vi "Ball Shooter Controller.vi"(8 "error in":errorcluster) -> ()   [LabVIEW 2016]
doc: "This VI executes continuously carrying out the current operation and responding to updates or new operations. It will often contain the timing or control code that is difficult to place directly in TeleOp. This VI generally opens all sensors and motors and isolates the rest of the robot code from knowing how the operations are carried out."
uses:
  Ball Shooter Setpoints.ctl
  Ball Shooter Operations.ctl
  <vilib>/Rock Robotics/WPI/ThirdParty/CanMotor/TalonSRX/WPI_CANTalonSRX_APIFeedbackSelect.ctl
  <vilib>/Rock Robotics/WPI/ThirdParty/CanMotor/TalonSRX/WPI_CANTalonSRX_APIControlMode.ctl
  <vilib>/Rock Robotics/WPI/SerialPort/WPI_SerialPort.ctl
  Ball Shooter Global.vi
panel:
  in  "Act":dbl
  out "Waveform Chart":cluster{"Act":dbl, "Encoder Velocity":dbl}(graph)
  in  "Cycle Period":dbl=1000.0
  in  "Cycle":bool
  out "Current\nCmd":string
  # "Tip: It may be helpful to observe inputs and sensor values.\nYou may also want to display tuning or debugging controls."
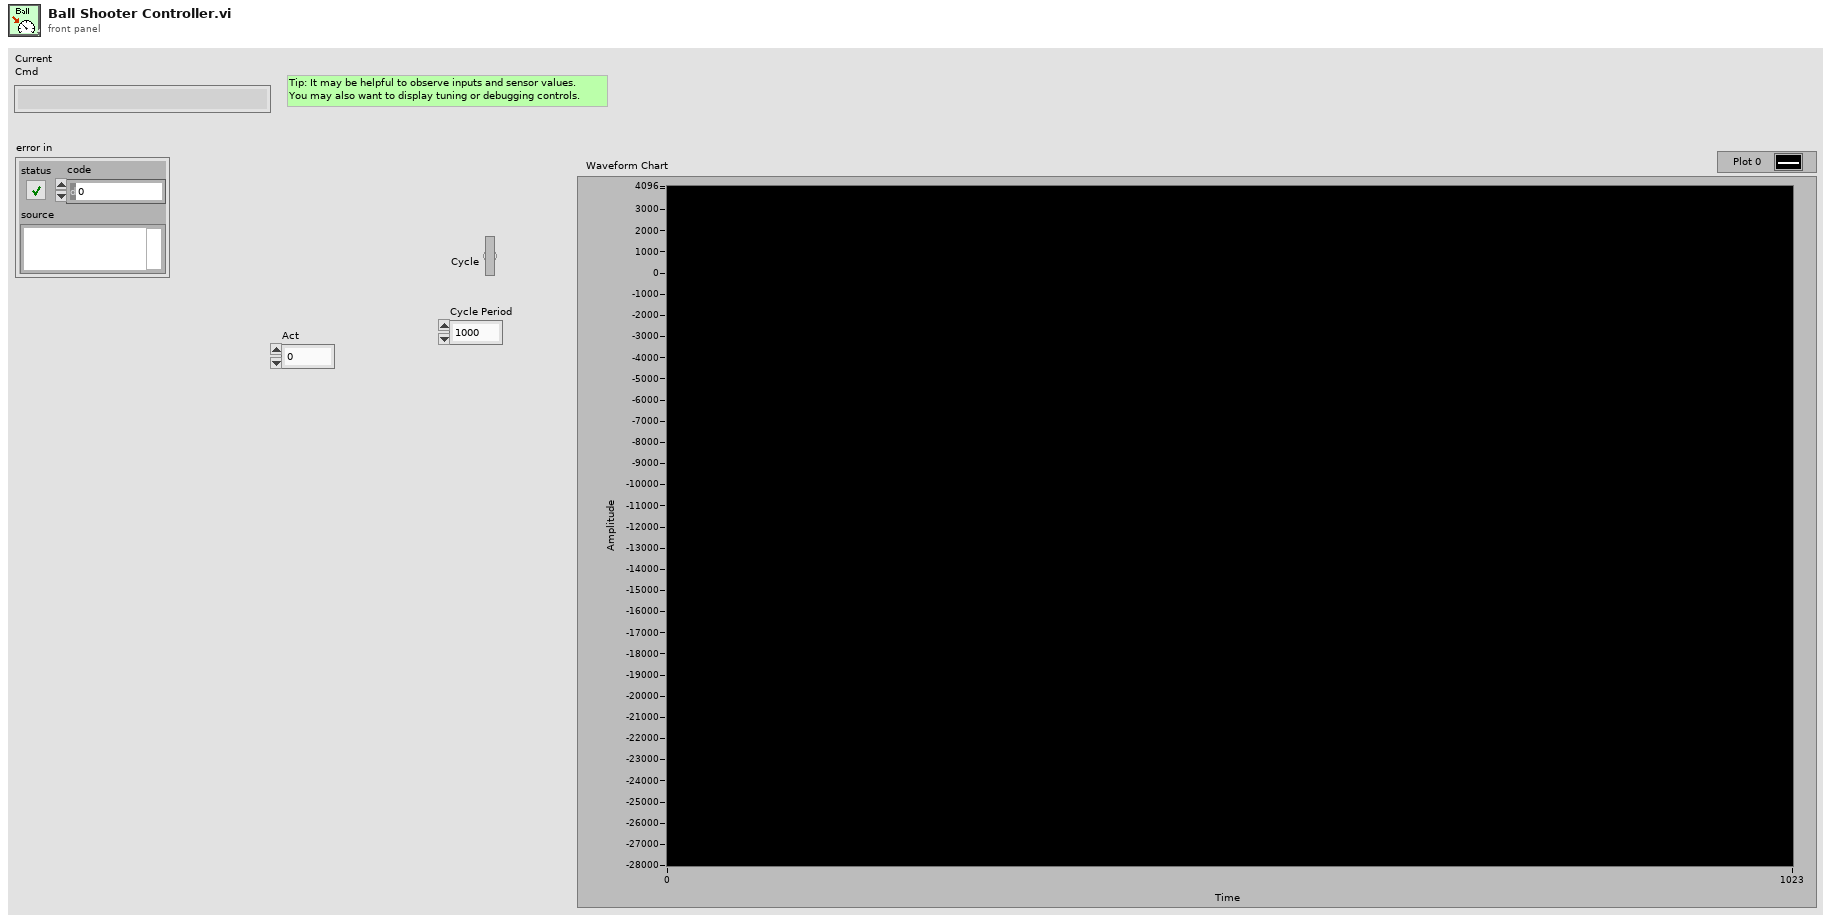
[diagram p1: front panel]
types:
  T1 = typedef "WPI_SerialPort.ctl" = enum16{"Onboard RS-232", "MXP TTL", "USB 1", "USB 2"}
  T2 = typedef "WPI_CANTalonSRX_APIControlMode.ctl" = enum8{"Percent VBus", "Speed", "Position", "Slave", "Unchanged / Invalid", "Voltage Compensation", "Current", "Motion Profile", "Motion Magic"}
  T3 = typedef "WPI_CANTalonSRX_APIFeedbackSelect.ctl" = enum16{"Digital Quadrature Encoder", "Analog Potentiometer", "Analog Encoder", "Count on Quad-A (Rising-Edge)", "Count on Quad-A (Falling-Edge)", "CTR Magnetic Enc (Absolute)", "CTR Magnetic Enc (Relative)", "Pulse Width"}
  T4 = typedef "Ball Shooter Setpoints.ctl" = cluster{"Operation":T5, "Setpoint":dbl, "Duration":dbl}
  T5 = typedef "Ball Shooter Operations.ctl" = enum16{"Reserve", "Read Current", "Immediate"}
  T6 = typedef "WPI_MotorControlDeviceRef.ctl" = cluster{"DeviceStatus":errorcluster, "Type":T7, "PWM":cluster{"PWM Channel":T8, "DeadBand":T9}, "CAN":cluster{"Device Number":u8, "SetOutput VI Ref":variant, "GetOutput VI Ref":variant, "Enable VI Ref":variant, "Disable VI Ref":variant, "Data":variant}, "Invert":bool}
  T7 = typedef "WPI_MotorControlType.ctl" = enum16{"PWM", "CAN"}
  T8 = typedef "FPGA_DIOPWMChannel.ctl" = enum8{"PWM 0", "PWM 1", "PWM 2", "PWM 3", "PWM 4", "PWM 5", "PWM 6", "PWM 7", "PWM 8", "PWM 9", "PWM MXP 0", "PWM MXP 1", "PWM MXP 2", "PWM MXP 3", "PWM MXP 4", "PWM MXP 5", "PWM MXP 6", "PWM MXP 7", "PWM MXP 8", "PWM MXP 9", "Invalid"}
  T9 = typedef "WPI_PWMDeadband.ctl" = cluster{"Name":string, "maxPositivePwm":i32, "minPositivePwm":i32, "centerPwm":i32, "maxNegativePwm":i32, "minNegativePwm":i32, "angularRange":u16}
  T10 = typedef "Command Status Info.ctl" = cluster{"Name":string, "Status":T11, "notifier out":T12}
  T11 = typedef "Completion Status.ctl" = enum16{"Successful", "Aborted", "Incomplete"}
  T12 = typedef "Completion Notifier.ctl" = refnum<notifier>
  T13 = cluster{"Default Command":T4, "Command Timing":cluster{"Start Time (ms)":u32, "Iterations":i32}, "Command Arguments":cluster{"Command Info":T10, "Description":string, "Default Command":T4, "notifier out":refnum<notifier>, "Subsystem Name":string}}
  T14 = typedef "WPI_SerialPortRef.ctl" = cluster{"DevStatus":errorcluster, "Serial Port Name":refnum<visa-resource-name>}
  T15 = typedef "WPI_CANTalonSRX_GlobalStatus.ctl" = cluster{"Applied Throttle":dbl, "Module Enabled":bool, "CAN Error":errorcluster, "Closed Loop Error":dbl, "Forward Limit Switch Closed":bool, "Reverse Limit Switch Closed":bool, "Sensor Position":dbl, "Sensor Velocity":dbl, "Current":dbl, "Sticky Fault - Over Temp":bool, "Sticky Fault - Under Voltage":bool, "Sticky Fault - Forward Limit":bool, "Sticky Fault - Reverse Limit":bool, "Sticky Fault - Forward Soft Limit":bool, "Sticky Fault - Reverse Soft Limit":bool, "Brake is Enabled":bool, "Encoder Position":dbl, "Encoder Velocity":dbl, "Encoder Index Count":dbl, "Encoder A Pin State":bool, "Encoder B Pin State":bool, "Encoder Index Pin State":bool, "Analog In":dbl, "Analog In Velocity":dbl, "Temperature (C)":dbl, "Battery Voltage":dbl, "Control 5 Is Supported":bool, "Current Profile Slot Select":dbl, "Pos Div 8":bool, "Vel Div 4":bool, "Pulse Width Position":i32, "Pulse Width Velocity":i32, "Pulse Width Rise To Rise (us)":i32, "Pulse Width Rise To Fall (us)":i32, "Mot Prof Active Is Under Run":bool, "Mot Prof Active Has Under Run":bool, "Mot Prof Active Is Last":bool, "Mot Prof Active Velocity Only":bool, "Mot Prof Active Is Valid":bool, "Mot Prof Buffer Is Full":bool, "Mot Prof Active Profile Slot Select":i32, "Mot Prof NextID":i32, "Mot Prof Count":i32, "Mot Prof Active Velocity":dbl, "Mot Prof Active Position":dbl, "Mot Prof Output Enable":i32}
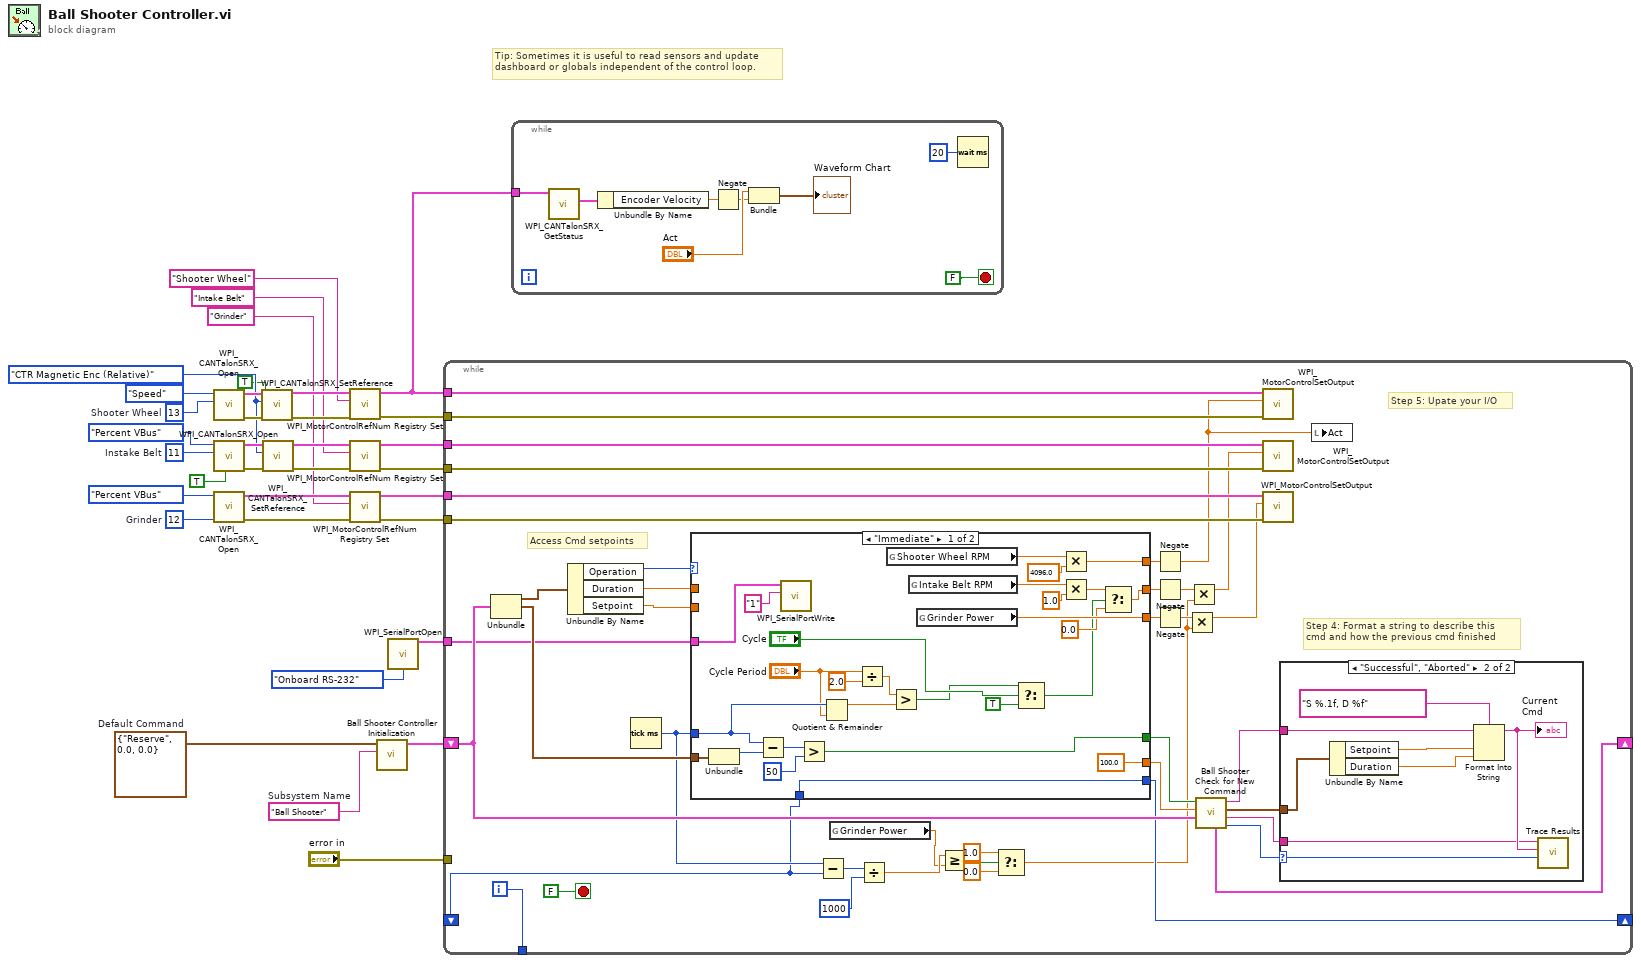
[diagram p0: block diagram]
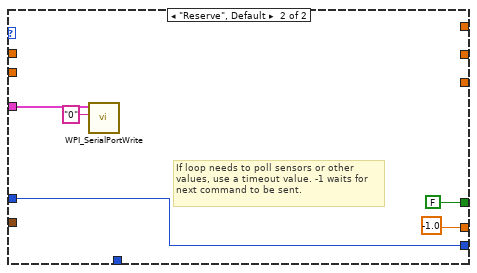
[diagram p3: hidden frame]
diagram:
  w21 = u8 12  # Grinder
  w23 = u8 11  # Instake Belt
  w24 = u8 13  # Shooter Wheel
  w26 = WPI_CANTalonSRX_APIFeedbackSelect."CTR Magnetic Enc (Relative)" ("Feedback Reference")
  w31 = T4 {"Operation"=enum."Reserve", "Setpoint"=0.0, "Duration"=0.0}  # Default Command
  w32 = "Ball Shooter"  # Subsystem Name
  # "Tip: Sometimes it is useful to read sensors and update\ndashboard or globals independent of the control loop."
  n1 = call <vilib>:"WPI_CANTalonSRX_Open.vi"("Device Number"=w24, "Control Mode"=WPI_CANTalonSRX_APIControlMode."Speed") -> ("error out"=w30:errorcluster, "CAN Talon SRX Ref"=w29:T6)  [unwired: 8 in]
  n2 = call <vilib>:"WPI_CANTalonSRX_Open.vi"("Invert"=TRUE, "Device Number"=w23, "Control Mode"=WPI_CANTalonSRX_APIControlMode."Percent VBus") -> ("error out"=w27:errorcluster, "CAN Talon SRX Ref"=w28:T6)  [unwired: 7 in]
  n3 = call <vilib>:"WPI_CANTalonSRX_Open.vi"("Device Number"=w21, "Control Mode"=WPI_CANTalonSRX_APIControlMode."Percent VBus") -> ("error out"=w12:errorcluster, "CAN Talon SRX Ref"=w14:T6)  [unwired: 8 in]
  n4 = call <vilib>:"WPI_CANTalonSRX_SetReference.vi"("error in (no error)"=w30, "Reverse Feedback Sensor"=TRUE, "Feedback Reference"=w26, "CAN Talon SRX Ref"=w29) -> ("error out"=w19:errorcluster, "CAN Talon SRX Ref"=w20:T6)  [unwired: 6 in]
  n5 = call <vilib>:"WPI_CANTalonSRX_SetReference.vi"("error in (no error)"=w27, "Feedback Reference"=w26, "CAN Talon SRX Ref"=w28) -> ("error out"=w11:errorcluster, "CAN Talon SRX Ref"=w16:T6)  [unwired: 7 in]
  n6 = call <vilib>:"WPI_MotorControlRefNum Registry Set.vi"("error in (no error)"=w19, "refnum name"="Shooter Wheel", "MotorControlDevRef"=w20) -> ("error out"=w17:errorcluster, "MotorControlDevRef"=w5:T6)  [unwired: 7 in]
  n7 = call <vilib>:"WPI_MotorControlRefNum Registry Set.vi"("error in (no error)"=w11, "refnum name"="Intake Belt", "MotorControlDevRef"=w16) -> ("error out"=w10:errorcluster, "MotorControlDevRef"=w15:T6)  [unwired: 7 in]
  n8 = call <vilib>:"WPI_MotorControlRefNum Registry Set.vi"("error in (no error)"=w12, "refnum name"="Grinder", "MotorControlDevRef"=w14) -> ("error out"=w9:errorcluster, "MotorControlDevRef"=w13:T6)  [unwired: 7 in]
  n9 = call "Ball Shooter Controller Initialization.vi"("Subsystem Name"=w32, "Default Command"=w31) -> ("Command Info"=w33:T13)  [unwired: 9 in]
  n10 = call <vilib>:"WPI_SerialPortOpen.vi"("Serial Port"=WPI_SerialPort."Onboard RS-232") -> ("SerialPortRef"=w2:T14)  [unwired: 13 in, 1 out]
  n11 = while {
    shift-right: [w67] -> _
    shift-left: w33 -> [w68]
    tunnel: [w74] -> _
    tunnel: "error in" -> [_]
    tunnel: w5 -> [w60]
    tunnel: w17 -> [w59]
    tunnel: w15 -> [w58]
    tunnel: w13 -> [w56]
    tunnel: w10 -> [w57]
    tunnel: w9 -> [w55]
    shift-right: [w47] -> _
    shift-left: _ -> [w48]
    tunnel: w2 -> [w35]
    i -> [w74]
    stop <- FALSE stop-if-true
    # "Step 5: Upate your I/O"
    # "Step 4: Format a string to describe this\ncmd and how the previous cmd finished"
    # "Access Cmd setpoints"
    n12 = Unbundle(w68) -> ("Default Command"=w73:T4, "Command Timing"=w70:cluster{"Start Time (ms)":u32, "Iterations":i32})  [unwired: 1 out]
    n13 = Unbundle By Name(w73) -> ("Operation"=w72:T5, "Duration"=w71:dbl, "Setpoint"=w69:dbl)
    n14 = Tick Count (ms)() -> (millisecond timer value=w49:u32)
    n15 = case shown="\"Immediate\"" w72 {
      tunnel: [100.0 -1.0] -> w65
      tunnel: [w105 FALSE ("ignore previous (F)")] -> w66
      tunnel: w70 -> [w106 _]
      tunnel: w71 -> [_ _]
      tunnel: w49 -> [w98 w113]
      tunnel: w69 -> [_ _]
      tunnel: [w99 _] -> w54
      tunnel: [w92 _] -> w53
      tunnel: [w104 _] -> w52
      tunnel: w48 -> [w86 _]
      tunnel: [w86 w113] -> w47
      tunnel: w35 -> [w85 w112]
      frame "Immediate" {
        n16 = Unbundle(w106) -> ("Start Time (ms)"=w109:u32)  [unwired: 1 out]
        n17 = Subtract(x=w98, y=w109) -> (x-y=w108:u32)
        n18 = call <vilib>:"WPI_SerialPortWrite.vi"("Buffer"="1", "SerialPortRef"=w85) -> ()  [unwired: 7 in, 3 out]
        n19 = Greater?(x=w108, y=u8 50 ("Left Motor")) -> (0:w105:bool)
        n20 = Quotient & Remainder(x=w98, y="Cycle Period") -> (x-y*floor(x/y)=w94:dbl)  [unwired: 1 out]
        n21 = Divide(x="Cycle Period", y=2.0) -> (x/y=w95:dbl)
        n22 = global read "Ball Shooter Global.vi" "Shooter Wheel RPM"() -> (w100:dbl)
        n23 = Greater?(x=w95, y=w94) -> (0:w88:bool)
        n24 = global read "Ball Shooter Global.vi" "Intake Belt RPM"() -> (w103:dbl)
        n25 = global read "Ball Shooter Global.vi" "Grinder Power"() -> (w104:dbl)
        n26 = Select(t=w88, s="Cycle", f=TRUE) -> (s? t:f=w90:bool)
        n27 = Multiply(x=w100, y=4096.0) -> (x*y=w99:dbl)
        n28 = Multiply(x=w103, y=1.0) -> (x*y=w93:dbl)
        n29 = Select(t=w93, s=w90, f=0.0) -> (s? t:f=w92:dbl)
      }
      frame "Reserve", Default {
        # "If loop needs to poll sensors or other\nvalues, use a timeout value. -1 waits for\nnext command to be sent."
        n30 = call <vilib>:"WPI_SerialPortWrite.vi"("Buffer"="0", "SerialPortRef"=w112) -> ()  [unwired: 7 in, 3 out]
      }
    }
    n31 = Subtract(x=w49, y=w48) -> (x-y=w46:u32)
    n32 = global read "Ball Shooter Global.vi" "Grinder Power"() -> (w43:dbl)
    n33 = Divide(x=w46, y=u32 1000) -> (x/y=w44:dbl)
    n34 = Greater Or Equal?(x=w44, y=w43) -> (x >= y?=w42:bool)
    n35 = Select(t=1.0, s=w42, f=0.0) -> (s? t:f=w36:dbl)
    n36 = Negate(x=w54) -> (-x=w50:dbl)
    n37 = Negate(x=w53) -> (-x=w51:dbl)
    n38 = Negate(x=w52) -> (-x=w38:dbl)
    n39 = Multiply(x=w38, y=w36) -> (x*y=w37:dbl)
    n40 = Multiply(x=w51, y=w36) -> (x*y=w39:dbl)
    n41 = call "Ball Shooter Check for New Command.vi"("Current Command"=w68, "Wait time (ms)"=w65, "Finished?"=w66) -> ("Completion"=w61:T11, "Subsystem Name"=w62:string, "Current Command"=w63:T4, "Initial Trace String"=w64:string, "NextCommand"=w67:T13)  [unwired: 4 in]
    n42 = call <vilib>:"WPI_MotorControlSetOutput.vi"("error in (no error)"=w59, "Output"=w50, "MotorControlDevRef"=w60) -> ()  [unwired: 6 in, 3 out]
    n43 = call <vilib>:"WPI_MotorControlSetOutput.vi"("error in (no error)"=w57, "Output"=w39, "MotorControlDevRef"=w58) -> ()  [unwired: 6 in, 3 out]
    n44 = call <vilib>:"WPI_MotorControlSetOutput.vi"("error in (no error)"=w55, "Output"=w37, "MotorControlDevRef"=w56) -> ()  [unwired: 6 in, 3 out]
    n45 = case shown="\"Successful\", \"Aborted\"" w61 {
      selector: w61 -> [_ w83]
      tunnel: w64 -> [_ w79]
      tunnel: w63 -> [_ w80]
      tunnel: w62 -> [_ w76]
      frame "Incomplete", Default {
        # "Continuing current command"
      }
      frame "Successful", "Aborted" {
        # "Report and setup for next command"
        n46 = Unbundle By Name(w80) -> ("Setpoint"=w82:dbl, "Duration"=w77:dbl)
        n47 = Format Into String(format string="S %.1f, D %f", initial string=w79, w82, w77) -> (resulting string=w78:string)  [unwired: 1 in, 1 out]
        "Current\nCmd" <- w78
        n48 = call <vilib>:"Trace Results.vi"("Status of previous command"=w83, "Description"=w78, "Subsystem"=w76) -> ()  [unwired: 9 in]
      }
    }
    n49 = local write "Act"(w50) -> ()
  }
  n50 = while {
    tunnel: w5 -> [w121]
    stop <- FALSE stop-if-true
    n51 = call <vilib>:"WPI_CANTalonSRX_GetStatus.vi"("CAN Talon SRX Ref"=w121) -> ("Talon SRX Status"=w120:T15)  [unwired: 8 in, 2 out]
    n52 = Unbundle By Name(w120) -> ("Encoder Velocity"=w119:dbl)
    n53 = Negate(x=w119) -> (-x=w116:dbl)
    n54 = Bundle("Act"="Act", w116) -> (→"Waveform Chart":cluster{"Act":dbl, dbl})  [unwired: 1 in]
    n55 = Wait (ms)(milliseconds to wait=u32 20) -> ()  [unwired: 1 out]
  }
